vi "Laurel Read All Active.vi"(6 "Connection Type":T1, 7 "VISA resource name":refnum<visa-resource-name>, 8 "error in (no error)":errorcluster, 10 "byte count in":i32=17, 11 "TCP Network Connection in":refnum<k5>) -> (0 "error out":errorcluster, 1 "trimmed string":string, 2 "Flow Rate (Item 1)":dbl, 3 "TCP Network Connection out":refnum<k5>, 4 "Gallons (Item 2)":dbl, 5 "VISA resource name 2":refnum<visa-resource-name>)   [LabVIEW 2016]
uses:
  Type Definitions/Laurel Connection Type.ctl
  <vilib>/Utility/error.llb/whitespace.ctl
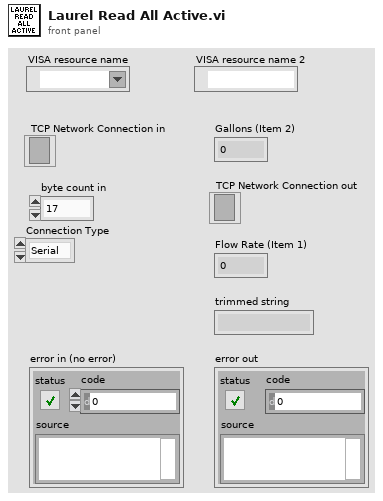
[diagram p1: front panel]
types:
  T1 = typedef "Laurel Connection Type.ctl" = enum16{"Serial", "TCP"}
  T2 = typedef "whitespace.ctl" = u16
  T3 = enum16{"Standard", "Buffered", "CRLF", "Immediate"}
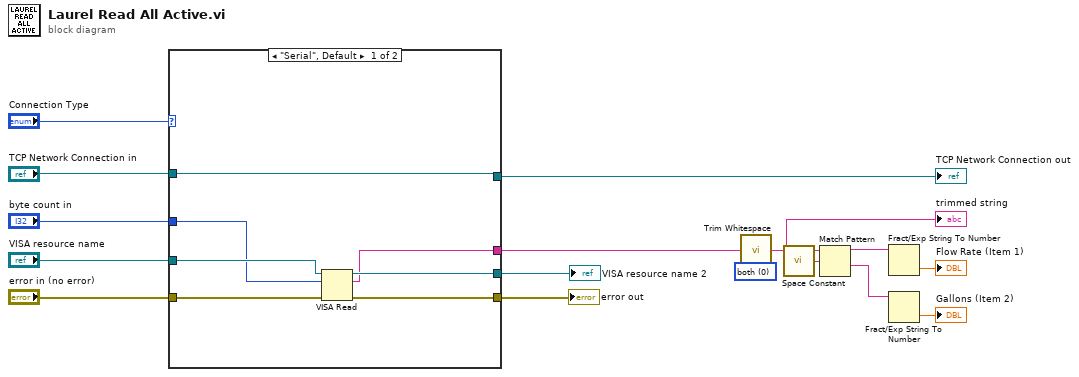
[diagram p0: block diagram]
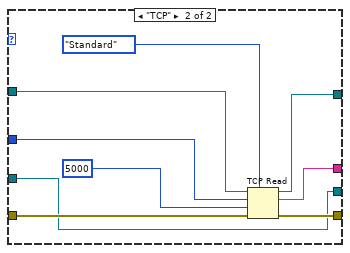
[diagram p2: hidden frame]
diagram:
  w6 = T2 0 items=["both", "start of string", "end of string"] ("location (both)")
  n1 = case shown="\"Serial\", Default" "Connection Type" {
    tunnel: "error in (no error)" -> [w22 w30]
    tunnel: [w23 w29] -> w9
    tunnel: [w18 w28] -> w8
    tunnel: [w21 w27] -> w7
    tunnel: "byte count in" -> [w17 w26]
    tunnel: "TCP Network Connection in" -> [w23 w25]
    tunnel: "VISA resource name" -> [w20 w24]
    tunnel: [w19 w24] -> w1
    frame "Serial", Default {
      n2 = VISA Read(VISA resource name=w20, byte count=w17, error in (no error)=w22) -> (VISA resource name out=w19:refnum<visa-resource-name>, read buffer=w18:string, error out=w21:errorcluster)  [unwired: 1 out]
    }
    frame "TCP" {
      n3 = TCP Read(connection ID=w25, bytes to read=w26, error in (no error)=w30, 7:T3."Standard" ("mode (standard)"), 9:5000 ("timeout ms (25000)")) -> (connection ID out=w29:refnum<k5>, data out=w28:string, error out=w27:errorcluster)
    }
  }
  "TCP Network Connection out" <- w9
  "error out" <- w7
  "VISA resource name 2" <- w1
  n4 = call <vilib>:"Trim Whitespace.vi"("string"=w8, "location (both)"=w6) -> ("trimmed string"=w14:string)
  "trimmed string" <- w14
  n5 = call <vilib>:"Space Constant.vi"() -> ("String"=w13:string)
  n6 = Match Pattern(string=w14, regular expression=w13) -> (before substring=w11:string, after substring=w12:string)  [unwired: 1 in, 2 out]
  n7 = Fract/Exp String To Number(string=w11) -> (number=→"Flow Rate (Item 1)":dbl)  [unwired: 3 in, 1 out]
  n8 = Fract/Exp String To Number(string=w12) -> (number=→"Gallons (Item 2)":dbl)  [unwired: 3 in, 1 out]
